vi "SVL Peak Sound Level.vi"   [LabVIEW 2017, in "SoundVib_SoundLevel.lvlib"]
doc: "Computes the peak sound level of <B>scaled signal [EU]</B>. <B>scaled signal [EU]</B> should have a zero DC component. You can attenuate the DC component with hardware AC-coupling filters and with software high-pass filters. The peak sound level is the maximum of the absolute values of all measured values. Wire data to the <B>scaled signal [EU]</B> input to determine the polymorphic instance to use or manually select the instance."
uses:
  <vilib>/addons/Sound and Vibration/svt_Level/SoundVib_SoundLevel.lvlib
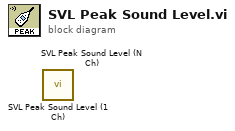
[diagram p0: block diagram]
diagram:
  n1 = call <vilib>:"SVL Peak Sound Level (1 Ch).vi"() -> ()  [unwired: 9 in, 3 out]
  n2 = call <vilib>:"SVL Peak Sound Level (N Ch).vi"() -> ()  [unwired: 9 in, 3 out]
